vi "DAQmx.Add Calibration to Devices.vi"(10 "Calibration in":T2(array[cluster]), 11 "Devices in":T1[](array[typedef])) -> (3 "Devices out":T1[](array[typedef]))   [LabVIEW 2019, in "DAQmx.lvclass"]
uses:
  DAQmx.lvclass
  typedefs/DeviceInfo--Cluster.ctl
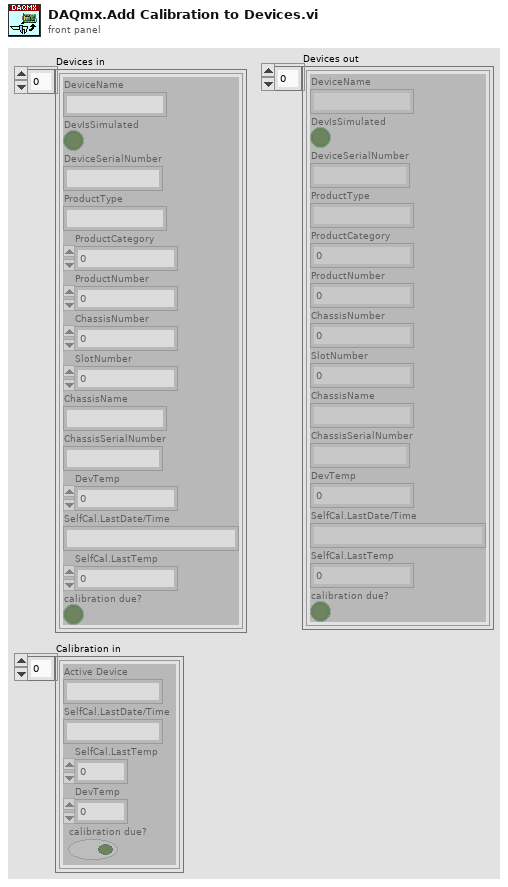
[diagram p1: front panel]
types:
  T1 = typedef "DAQmx.lvclass/DeviceInfo--Cluster.ctl" = cluster{"DeviceName":string, "DevIsSimulated":bool, "DeviceSerialNumber":string, "ProductType":string, "ProductCategory":i32, "ProductNumber":u32, "ChassisNumber":u32, "SlotNumber":u32, "ChassisName":string, "ChassisSerialNumber":string, "DevTemp":dbl, "SelfCal.LastDate/Time":string, "SelfCal.LastTemp":dbl, "calibration due?":bool}
  T2 = cluster{"Active Device":string, "SelfCal.LastDate/Time":string, "SelfCal.LastTemp":dbl, "DevTemp":dbl, "calibration due?":bool}[]
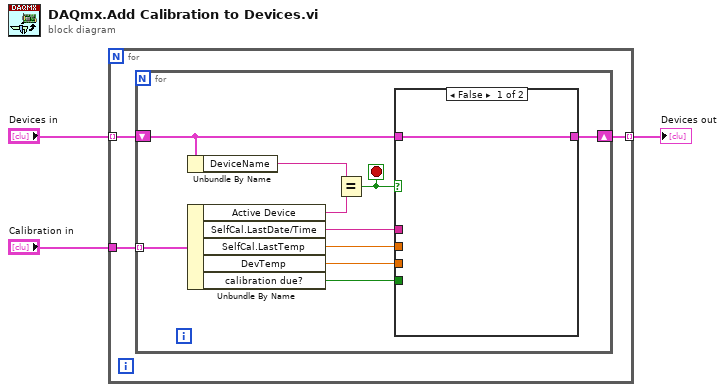
[diagram p0: block diagram]
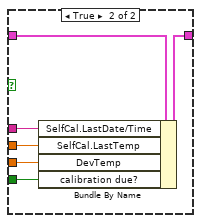
[diagram p2: hidden frame]
diagram:
  n1 = for {
    tunnel: "Devices in" -> [w6] mode=indexing
    tunnel: "Calibration in" -> [w5]
    tunnel: [w4] -> w3 mode=indexing
    n2 = for {
      tunnel: w5 -> [w12] mode=indexing
      shift-right: [w10] -> w4
      shift-left: w6 -> [w11]
      stop <- w9 stop-if-true
      n3 = Unbundle By Name(w11) -> ("DeviceName"=w8:string)
      n4 = Unbundle By Name(w12) -> ("Active Device"=w7:string, "SelfCal.LastDate/Time"=w15:string, "SelfCal.LastTemp"=w16:dbl, "DevTemp"=w14:dbl, "calibration due?"=w13:bool)
      n5 = Equal?(x=w8, y=w7) -> (x = y?=w9:bool)
      n6 = case shown="False" w9 {
        tunnel: w11 -> [w17 w19]
        tunnel: w16 -> [_ w23]
        tunnel: w15 -> [_ w22]
        tunnel: w14 -> [_ w21]
        tunnel: w13 -> [_ w20]
        tunnel: [w17 w18] -> w10
        frame False {
        }
        frame True {
          n7 = Bundle By Name(cluster=w19, "SelfCal.LastDate/Time"=w22, "SelfCal.LastTemp"=w23, "DevTemp"=w21, "calibration due?"=w20) -> (w18:T1)
        }
      }
    }
  }
  "Devices out" <- w3
